vi "Error Handler.vi"(8 "error in (no error)":errorcluster, 9 "ClearCommandError (false)":bool, 10 "ClearDeviceError (false)":bool, 11 "VISA resource name":refnum<visa-resource-name>) -> (0 "error out":errorcluster, 1 "IsCommandError":bool, 2 "device error out":errorcluster, 3 "VISA resource name out":refnum<visa-resource-name>)   [LabVIEW 2015, in "JULABO DeviceDriver.lvlib"]
doc: "Checks whether the error in the error cluster is an device specific error and checks whether device has an alarm or a warning."
uses:
  JULABO DeviceDriver.lvlib
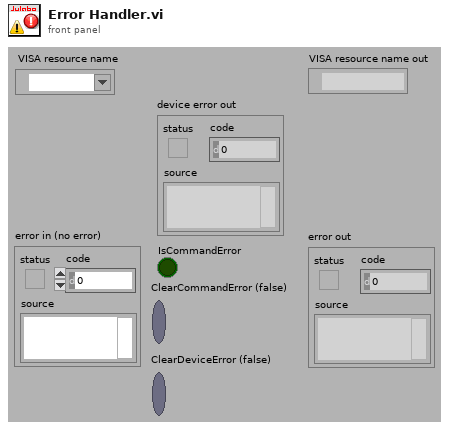
[diagram p1: front panel]
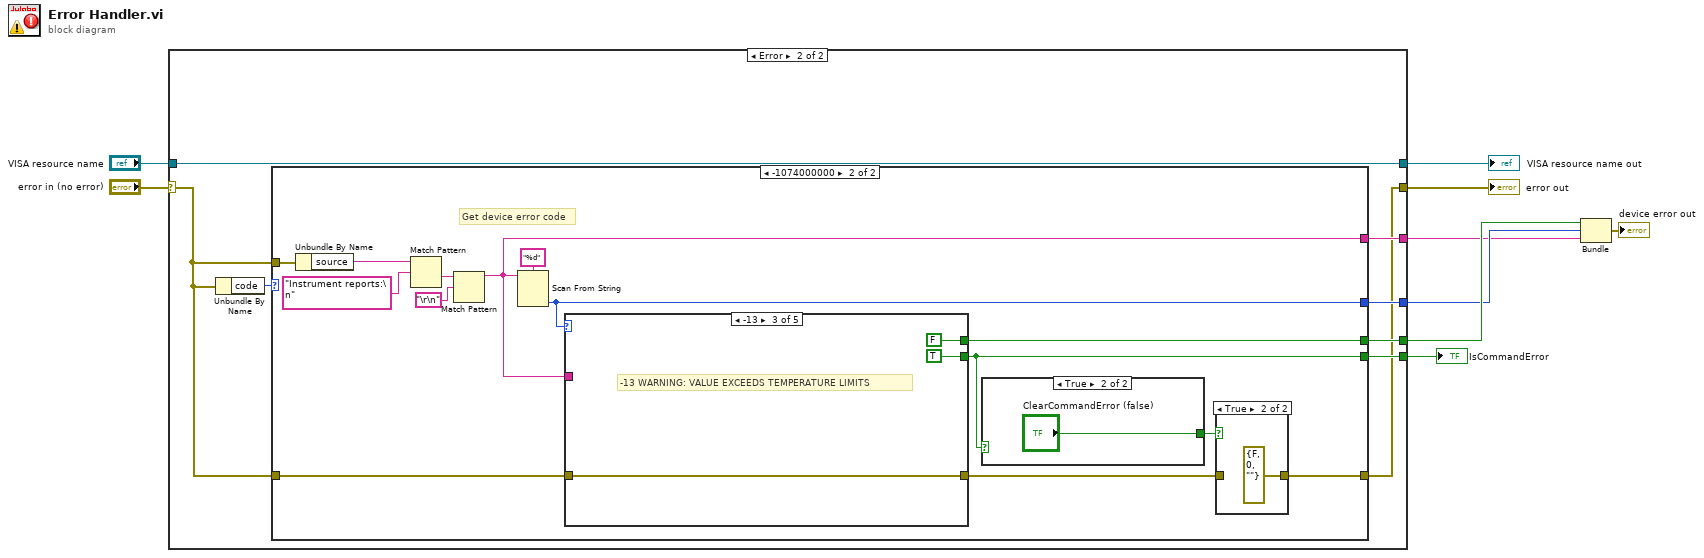
[diagram p0: block diagram]
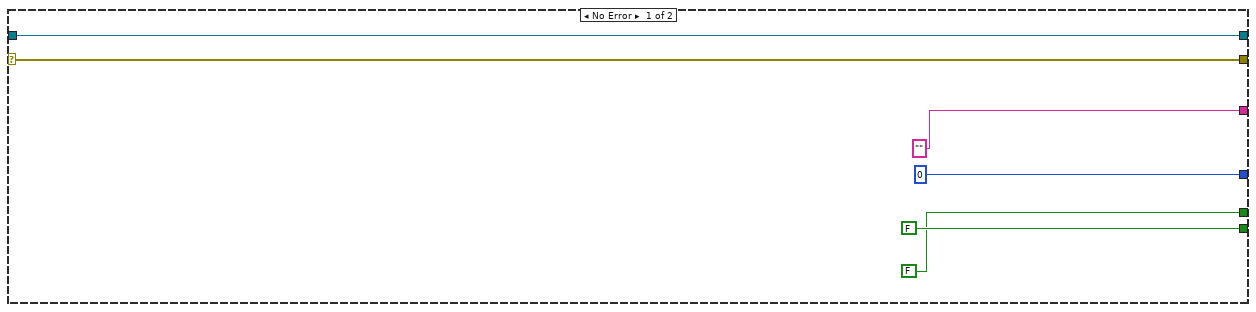
[diagram p2: hidden frame]
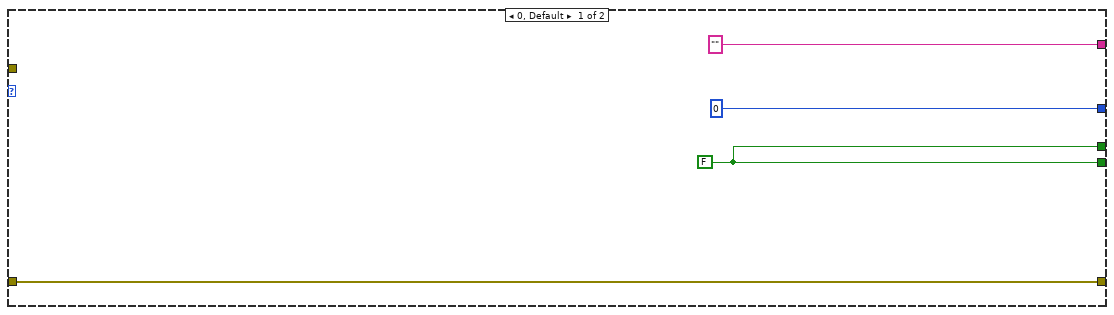
[diagram p3: hidden frame]
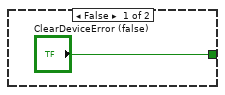
[diagram p5: hidden frame]
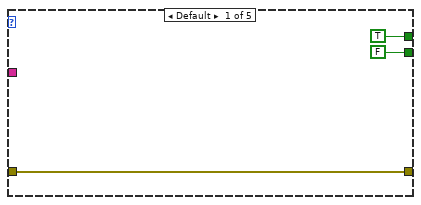
[diagram p6: hidden frame]
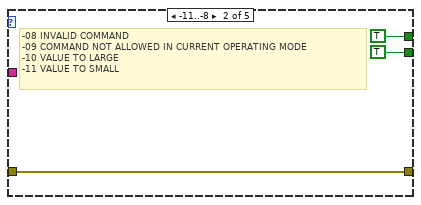
[diagram p7: hidden frame]
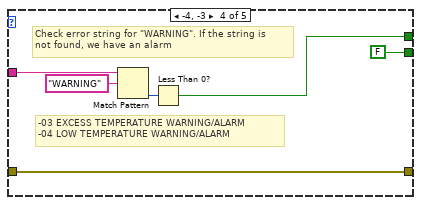
[diagram p8: hidden frame]
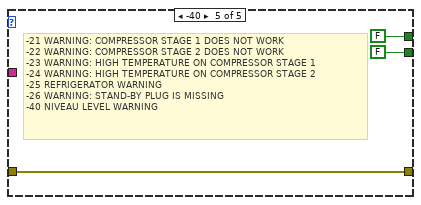
[diagram p9: hidden frame]
diagram:
  n1 = case shown="Error" "error in (no error)" {
    selector: "error in (no error)" -> [w15 w17]
    tunnel: [w14 w23] -> w9
    tunnel: "VISA resource name" -> [w14 w23]
    tunnel: [w15 w18] -> w7
    tunnel: ["" w22] -> w2
    tunnel: [0 w21] -> w3
    tunnel: [FALSE w20] -> w5
    tunnel: [FALSE w19] -> w4
    frame No Error {
    }
    frame Error {
      n2 = Unbundle By Name(w17) -> ("code"=w16:i32)
      n3 = case shown="-1074000000" w16 {
        tunnel: w17 -> [_ w41]
        tunnel: ["" w33] -> w22
        tunnel: [0 w35] -> w21
        tunnel: [w24 w32] -> w20
        tunnel: [w24 w34] -> w19
        tunnel: [w25 w30] -> w18
        tunnel: w17 -> [w25 w28]
        frame 0, Default {
          w24 = FALSE
        }
        frame -1074000000 {
          # "Get device error code"
          n4 = Unbundle By Name(w41) -> ("source"=w40:string)
          n5 = Match Pattern(string=w40, regular expression="Instrument reports:\n" ("String")) -> (after substring=w37:string)  [unwired: 1 in, 3 out]
          n6 = Match Pattern(string=w37, regular expression="\r\n") -> (before substring=w33:string)  [unwired: 1 in, 3 out]
          n7 = Scan From String(format string="%d" ("Format-String"), input string=w33) -> (output 1=w35:i32)  [unwired: 3 in, 3 out]
          n8 = case shown="-13" w35 {
            tunnel: [FALSE TRUE TRUE FALSE FALSE] -> w32
            tunnel: w33 -> [_ _ _ w60 _]
            tunnel: [TRUE TRUE FALSE w57 FALSE] -> w34
            tunnel: [w46 w49 w52 w55 w61] -> w31
            tunnel: w28 -> [w46 w49 w52 w55 w61]
            frame Default {
            }
            frame -11..-8 {
              # "-08 INVALID COMMAND\n-09 COMMAND NOT ALLOWED IN CURRENT OPERATING MODE\n-10 VALUE TO LARGE\n-11 VALUE TO SMALL"
            }
            frame -13 {
              # "-13 WARNING: VALUE EXCEEDS TEMPERATURE LIMITS"
            }
            frame -4, -3 {
              # "Check error string for \"WARNING\". If the string is\nnot found, we have an alarm"
              # "-03 EXCESS TEMPERATURE WARNING/ALARM\n-04 LOW TEMPERATURE WARNING/ALARM"
              n9 = Match Pattern(string=w60, regular expression="WARNING" ("regulärer Ausdruck")) -> (offset past match=w58:i32)  [unwired: 1 in, 3 out]
              n10 = Less Than 0?(x=w58) -> (x < 0?=w57:bool)
            }
            frame -40 {
              # "-21 WARNING: COMPRESSOR STAGE 1 DOES NOT WORK\n-22 WARNING: COMPRESSOR STAGE 2 DOES NOT WORK\n-23 WARNING: HIGH TEMPERATURE ON COMPRESSOR STAGE 1\n-24 WARNING: HIGH TEMPERATURE ON COMPRESSOR STAGE 2\n-25 REFRIGERATOR WARNING\n-26 WARNING: STAND-BY PLUG IS MISSING\n-40 NIVEAU LEVEL WARNING"
            }
          }
          n11 = case shown="True" w32 {
            tunnel: ["ClearDeviceError (false)" "ClearCommandError (false)"] -> w29
            frame False {
            }
            frame True {
            }
          }
          n12 = case shown="True" w29 {
            tunnel: [w42 errorcluster {"status"=FALSE, "code"=0, "source"=""} ("error IO")] -> w30
            tunnel: w31 -> [w42 _]
            frame False {
            }
            frame True {
            }
          }
        }
      }
    }
  }
  "VISA resource name out" <- w9
  "error out" <- w7
  "IsCommandError" <- w5
  n13 = Bundle(w4, w3, "source"=w2) -> (→"device error out":cluster{bool, i32, "source":string})  [unwired: 1 in]
